vi "FloorplanFromOBJfile.vi"() -> ()   [LabVIEW 2022 SP3]
uses:
  Instance           1 28Saved   FloorplanFromOBJfile .vi
panel:
  out "FloorplanArray":T1(array[cluster]) {"zNorm" format="%.2f"; "yNorm" format="%.2f"; "xNorm" format="%.2f"; "zVert" format="%^#_6g"; "yVert" format="%^#_6g"; "xVert" format="%^#_6g"}
  # "Run, and point it at an OBJ file..."
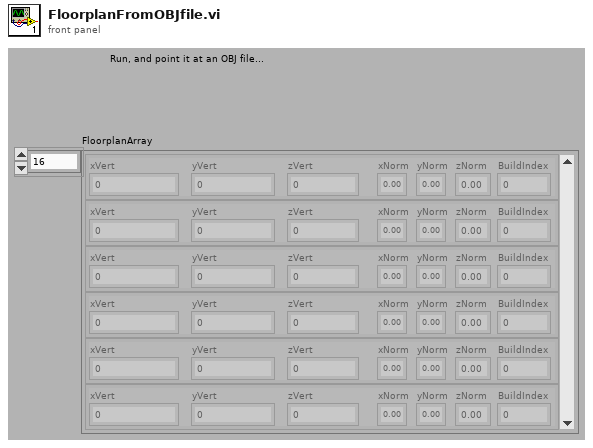
[diagram p1: front panel]
types:
  T1 = cluster{"xVert":dbl, "yVert":dbl, "zVert":dbl, "xNorm":dbl, "yNorm":dbl, "zNorm":dbl, "BuildIndex":u32}[]
  T2 = cluster{"BuildAverage":cluster{"x":dbl, "y":dbl, "z":dbl}, "BuildIndex":u32, "BuildMax":cluster{"x":dbl, "y":dbl, "z":dbl}, "BuildMin":cluster{"x":dbl, "y":dbl, "z":dbl}}[]
  T3 = cluster{"BuildAverage":cluster{"x":dbl, "y":dbl, "z":dbl}, "BuildIndex":u32, "BuildMax":cluster{"x":dbl, "y":dbl, "z":dbl}, "BuildMin":cluster{"x":dbl, "y":dbl, "z":dbl}}
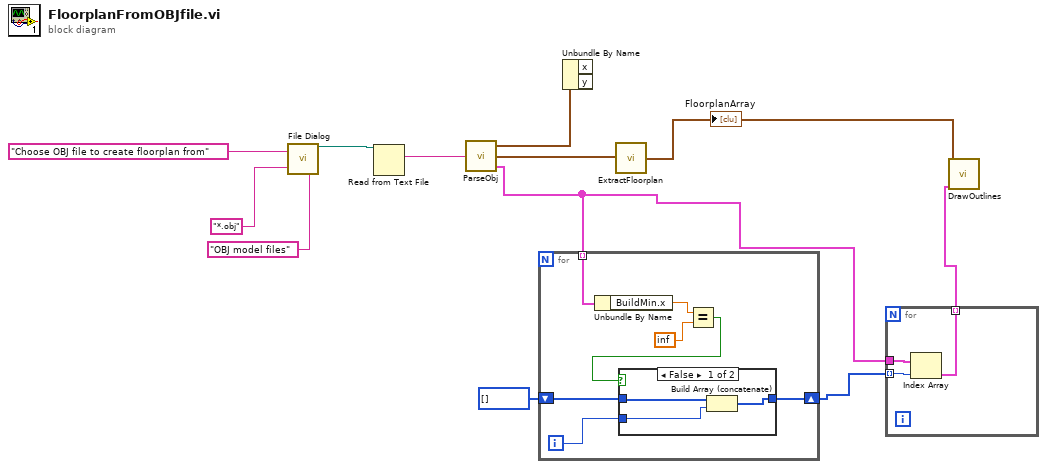
[diagram p0: block diagram]
diagram:
  n1 = call "File Dialog"("prompt"="Choose OBJ file to create floorplan from", "pattern (all files)"="*.obj", "pattern label"="OBJ model files") -> ("selected path"=w10:path)  [unwired: 4 in, 8 out]
  n2 = Read from Text File(file (use dialog)=w10) -> (text=w11:string)  [unwired: 1 in, 5 out]
  n3 = call "ParseObj.vi"("String"=w11) -> ("BuildingInfoArray"=w2:T2, "FaceArray"=w12:T1, "SiteAverage"=w5:cluster{"x":dbl, "y":dbl, "z":dbl})  [unwired: 2 out]
  n4 = for {
    tunnel: w2 -> [w19] mode=indexing
    shift-right: [w15] -> w3
    shift-left: i32[] [] -> [w14]
    i -> [w13]
    n5 = Unbundle By Name(w19) -> ("BuildMin.x"=w18:dbl)
    n6 = Equal?(x=w18, y=inf) -> (x = y?=w16:bool)
    n7 = case shown="False" w16 {
      tunnel: [w21 w23] -> w15
      tunnel: w14 -> [w22 w23]
      tunnel: w13 -> [w20 _]
      frame False {
        n8 = Build Array (concatenate)(w22, w20) -> (w21:i32[])
      }
      frame True {
      }
    }
  }
  n9 = Unbundle By Name(w5) -> ()  [unwired: 2 out]
  n10 = call "ExtractFloorplan.vi"("FaceArray"=w12) -> ("FloorplanArray"=w6:T1)  [unwired: 4 out]
  "FloorplanArray" <- w6
  n11 = for {
    tunnel: w3 -> [w26] mode=indexing
    tunnel: w2 -> [w25]
    tunnel: [w24] -> w1 mode=indexing
    n12 = Index Array(array=w25, index=w26) -> (element=w24:T3)
  }
  n13 = call "DrawOutlines.vi"("BuildingInfoArray"=w1, "FloorplanArray"=w6) -> ()  [unwired: 2 in, 8 out]
